vi "Launch IO Trace.vi"(7 "error in (no error)":errorcluster, 9 "launch method (standard)":T1(ring)) -> (0 "error out":errorcluster)   [LabVIEW 2010, in "NI IO Trace.lvlib"]
doc: "Launches NI I/O Trace if it isn't current running.\n\n<b>Note:</b> Only one instance of NI I/O Trace may be running at a time"
uses:
  <vilib>/NiIOTrace/NI IO Trace.lvlib
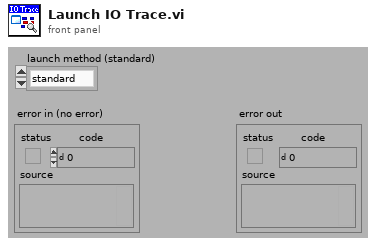
[diagram p1: front panel]
types:
  T1 = enum16{"standard", "maximized", "minimized", "hidden"}
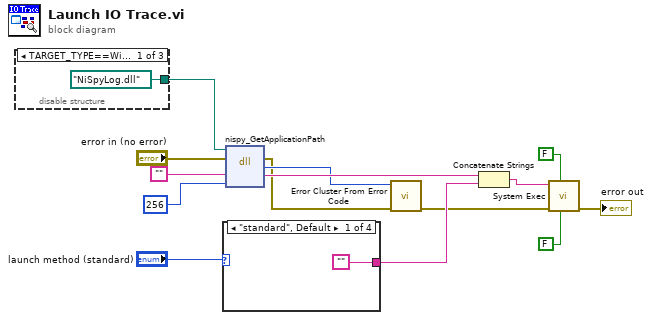
[diagram p0: block diagram]
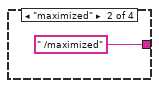
[diagram p2: hidden frame]
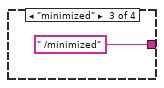
[diagram p3: hidden frame]
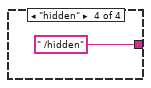
[diagram p4: hidden frame]
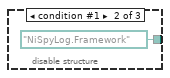
[diagram p5: hidden frame]
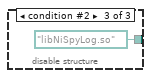
[diagram p6: hidden frame]
diagram:
  n1 = disable-structure shown="TARGET_TYPE==Windows, default" {
    disable-tunnel: [path "NiSpyLog.dll" ("path in") path "NiSpyLog.Framework" ("path in") path "libNiSpyLog.so" ("path in")] -> w12
    frame condition #0 (active) {
    }
    frame condition #1 {
    }
    frame condition #2 {
    }
  }
  n2 = case shown="\"standard\", Default" "launch method (standard)" {
    tunnel: ["" " /maximized" " /minimized" ("string") " /hidden" ("string")] -> w6
    frame "standard", Default {
    }
    frame "maximized" {
    }
    frame "minimized" {
    }
    frame "hidden" {
    }
  }
  n3 = dll-call lib="C:/WINDOWS/system32/NiSpyLog.dll" fn="nispy_GetApplicationPath" label="GetSpyApplicationPathname"(path in=w12, error in="error in (no error)", "path"="", "length"=256 ("dimension size")) -> (error out=w5:errorcluster, "return type"=w8:i32, "path"=w10:string)  [unwired: 2 in, 1 out]
  n4 = call <vilib>:"Error Cluster From Error Code.vi"("error in (no error)"=w5, "error code (0)"=w8) -> ("error out"=w4:errorcluster)  [unwired: 1 in, 6 out]
  n5 = Concatenate Strings(w10, w6) -> (w1:string)
  n6 = call <vilib>:"System Exec.vi"("run minimized? (F)"=FALSE, "wait until completion? (T)"=FALSE, "error in (no error)"=w4, "command line"=w1) -> ("error out"=→"error out":errorcluster)  [unwired: 2 in, 5 out]
